vi "8 Bit Cluster to 64 Bit Element (SubVI).vi"(11 "Pixel Cluster":T1) -> (3 "Pixel Data (64-Bit)":u64)   [LabVIEW 2015]
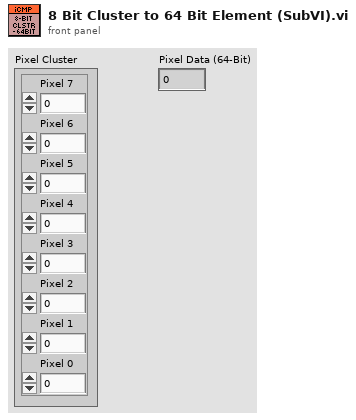
[diagram p1: front panel]
types:
  T1 = cluster{"Pixel 7":u8, "Pixel 6":u8, "Pixel 5":u8, "Pixel 4":u8, "Pixel 3":u8, "Pixel 2":u8, "Pixel 1":u8, "Pixel 0":u8}
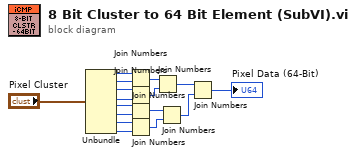
[diagram p0: block diagram]
diagram:
  n1 = Unbundle("Pixel Cluster") -> ("Pixel 7"=w3:u8, "Pixel 6"=w2:u8, "Pixel 5"=w4:u8, "Pixel 4"=w5:u8, "Pixel 3"=w6:u8, "Pixel 2"=w7:u8, "Pixel 1"=w8:u8, "Pixel 0"=w9:u8)
  n2 = Join Numbers(hi=w3, lo=w2) -> ((hi.lo)=w13:u16)
  n3 = Join Numbers(hi=w4, lo=w5) -> ((hi.lo)=w14:u16)
  n4 = Join Numbers(hi=w6, lo=w7) -> ((hi.lo)=w15:u16)
  n5 = Join Numbers(hi=w8, lo=w9) -> ((hi.lo)=w10:u16)
  n6 = Join Numbers(hi=w13, lo=w14) -> ((hi.lo)=w11:u32)
  n7 = Join Numbers(hi=w15, lo=w10) -> ((hi.lo)=w12:u32)
  n8 = Join Numbers(hi=w11, lo=w12) -> ((hi.lo)=→"Pixel Data (64-Bit)":u64)
